vi "PLC.Dial800.OPC Connect.vi"(8 "error in (no error)":errorcluster, 9 "ms timeout (1000)":i32, 11 "Var URLs In":T1[](array[typedef])) -> (0 "error out":errorcluster, 3 "Var URLs":T1[](array[typedef]))   [LabVIEW 2018]
uses:
  PLC.Dial800.Var URL Item.ctl
  PLC.Dial800.VarNameSelector.ctl
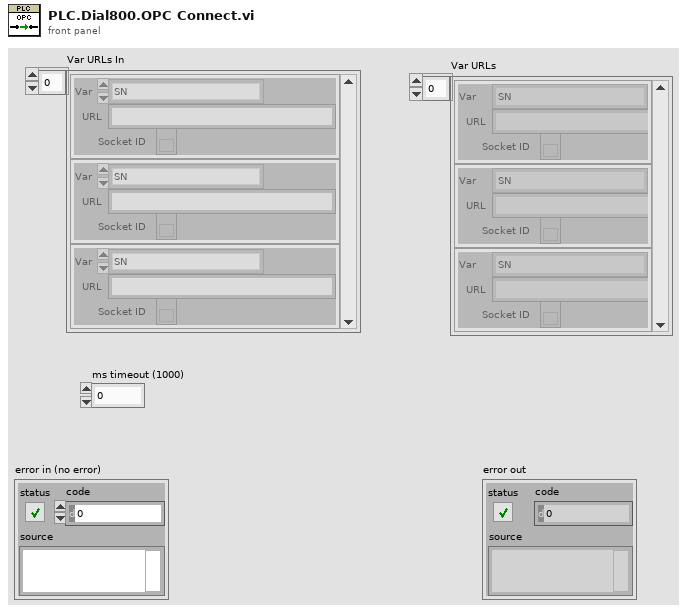
[diagram p1: front panel]
types:
  T1 = typedef "PLC.Dial800.Var URL Item.ctl" = cluster{"Var":T2, "URL":string, "Socket ID":refnum<k13>}
  T2 = typedef "PLC.Dial800.VarNameSelector.ctl" = enum16{"SN", "Reset", "HeartBeat_PLC", "Heartbeat_PC", "Start", "Running", "Done", "Pass"}
  T3 = enum16{"Read", "Write", "ReadWrite", "BufferedRead", "BufferedReadWrite"}
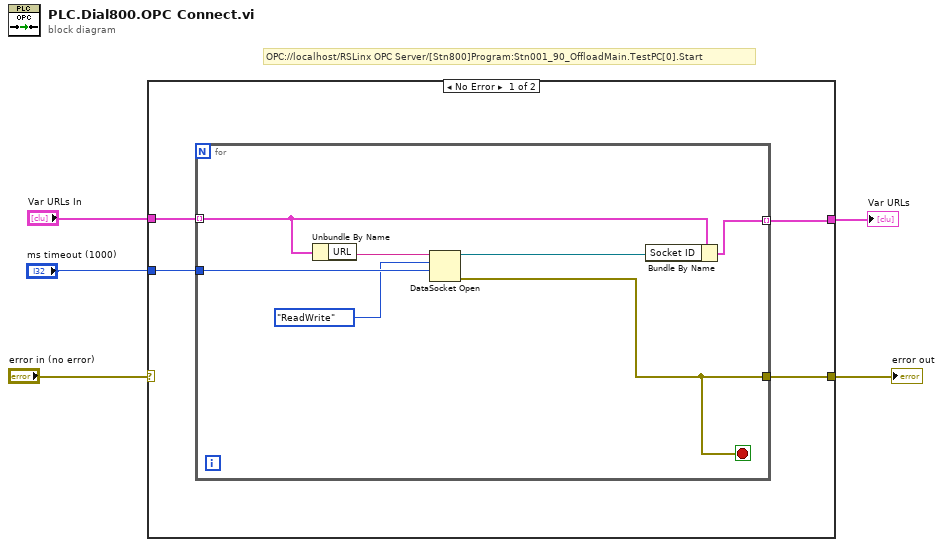
[diagram p0: block diagram]
diagram:
  # "OPC://localhost/RSLinx OPC Server/[Stn800]Program:Stn001_90_OffloadMain.TestPC[0].Start"
  n1 = case shown="No Error" "error in (no error)" {
    selector: "error in (no error)" -> [_ w18]
    tunnel: [w9 w18] -> w4
    tunnel: [w7 w17] -> w3
    tunnel: "Var URLs In" -> [w8 w17]
    tunnel: "ms timeout (1000)" -> [w6 _]
    frame No Error {
      n2 = for {
        tunnel: [w10] -> w9
        tunnel: w8 -> [w15] mode=indexing
        tunnel: [w13] -> w7 mode=indexing
        tunnel: w6 -> [w12]
        stop <- w10 stop-if-true
        n3 = Unbundle By Name(w15) -> ("URL"=w14:string)
        n4 = DataSocket Open(9:w12, 10:T3."ReadWrite" ("mode"), 11:w14) -> (0:w10:errorcluster, 3:w16:refnum<k13>)  [unwired: 1 in]
        n5 = Bundle By Name(cluster=w15, "Socket ID"=w16) -> (w13:T1)
      }
    }
    frame Error {
    }
  }
  "error out" <- w4
  "Var URLs" <- w3
